vi "Check Errors.vi"(8 "error in (no error)":errorcluster, 11 "standard error":string) -> (0 "error out":errorcluster)   [LabVIEW 2013, in "PL Framework Configuration Tool.lvlib" / "SCP File Transfer.lvclass"]
uses:
  SCP File Transfer.lvclass
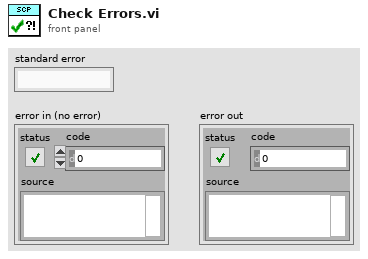
[diagram p1: front panel]
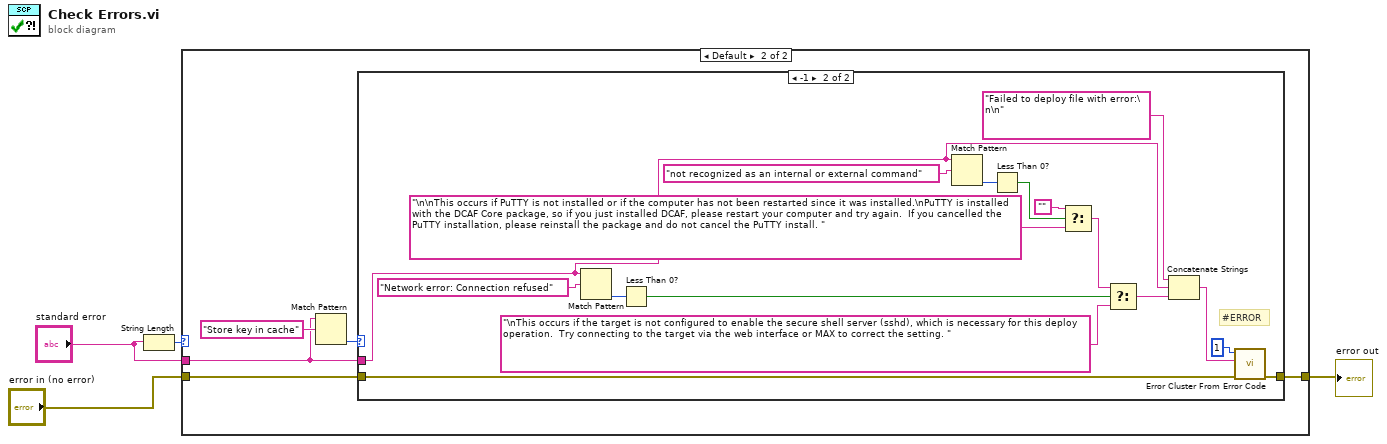
[diagram p0: block diagram]
diagram:
  n1 = String Length(string="standard error") -> (length=w1:i32)
  n2 = case shown="Default" w1 {
    tunnel: "standard error" -> [_ w7]
    tunnel: "error in (no error)" -> [w5 w10]
    tunnel: [w5 w9] -> w4
    frame 0 {
    }
    frame Default {
      n3 = Match Pattern(string=w7, regular expression="Store key in cache") -> (offset past match=w6:i32)  [unwired: 1 in, 3 out]
      n4 = case shown="-1" w6 {
        tunnel: w10 -> [w11 w28]
        tunnel: [w11 w27] -> w9
        tunnel: w7 -> [_ w18]
        frame Default {
          # "This is an error message that is automatically handled by the 'echo y | prefix, due to the credentials for that target not being stored in the credential cache yet.  Don't scare a user with this expected error, suppress it and move on."
        }
        frame -1 {
          # "#ERROR"
          n5 = Match Pattern(string=w18, regular expression="Network error: Connection refused") -> (offset past match=w16:i32)  [unwired: 1 in, 3 out]
          n6 = Less Than 0?(x=w16) -> (x < 0?=w15:bool)
          n7 = Match Pattern(string=w18, regular expression="not recognized as an internal or external command") -> (offset past match=w21:i32)  [unwired: 1 in, 3 out]
          n8 = Less Than 0?(x=w21) -> (x < 0?=w22:bool)
          n9 = Select(t="", s=w22, f="\n\nThis occurs if PuTTY is not installed or if the computer has not been restarted since it was installed.\nPuTTY is installed with the DCAF Core package, so if you just installed DCAF, please restart your computer and try again.  If you cancelled the PuTTY installation, please reinstall the package and do not cancel the PuTTY install. ") -> (s? t:f=w14:string)
          n10 = Select(t=w14, s=w15, f="\nThis occurs if the target is not configured to enable the secure shell server (sshd), which is necessary for this deploy operation.  Try connecting to the target via the web interface or MAX to correct the setting. ") -> (s? t:f=w12:string)
          n11 = Concatenate Strings("Failed to deploy file with error:\n\n" ("string"), w18, w12) -> (w25:string)
          n12 = call <vilib>:"Error Cluster From Error Code.vi"("error in (no error)"=w28, "error message (\"\")"=w25, "error code (0)"=1) -> ("error out"=w27:errorcluster)  [unwired: 6 in]
        }
      }
    }
  }
  "error out" <- w4
